vi "Launch System uServices.vi"(8 "error in (no error)":errorcluster, 11 "Guardian in":refnum<class "Guardian.lvclass">) -> (0 "error out":errorcluster, 3 "Guardian out":refnum<class "Guardian.lvclass">)   [LabVIEW 2026, in "TALOS.lvlib" / "Guardian.lvlib" / "Guardian.lvclass"]
uses:
  Guardian.lvclass
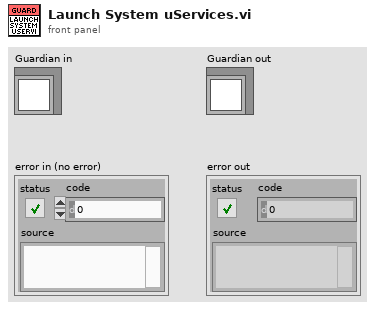
[diagram p1: front panel]
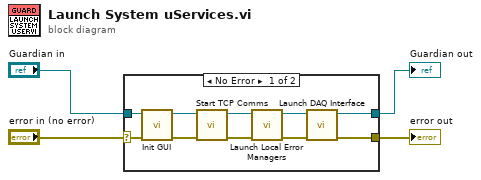
[diagram p0: block diagram]
diagram:
  n1 = case shown="No Error" "error in (no error)" {
    selector: "error in (no error)" -> [w14 w16]
    tunnel: "Guardian in" -> [w13 w15]
    tunnel: [w9 w16] -> w2
    tunnel: [w10 w15] -> w1
    frame No Error {
      n2 = call "Init GUI.vi"("error in (no error)"=w14, "Guardian in"=w13) -> ("error out"=w12:errorcluster, "Guardian out"=w11:refnum<class "Guardian.lvclass">)  [unwired: 8 in]
      n3 = call "Start TCP Comms.vi"("error in (no error)"=w12, "Guardian in"=w11) -> ("error out"=w7:errorcluster, "Guardian out"=w8:refnum<class "Guardian.lvclass">)  [unwired: 8 in]
      n4 = call "Launch Local Error Managers.vi"("error in (no error)"=w7, "Guardian in"=w8) -> ("error out"=w5:errorcluster, "Guardian out"=w6:refnum<class "Guardian.lvclass">)  [unwired: 8 in]
      n5 = call "Launch DAQ Interface.vi"("error in (no error)"=w5, "Guardian in"=w6) -> ("error out"=w9:errorcluster, "Guardian out"=w10:refnum<class "Guardian.lvclass">)  [unwired: 8 in]
    }
    frame Error {
    }
  }
  "error out" <- w2
  "Guardian out" <- w1
